vi "Append_Suffiix.vi"(1 "Results file":path) -> (0 "appended path":path)   [LabVIEW 2020]
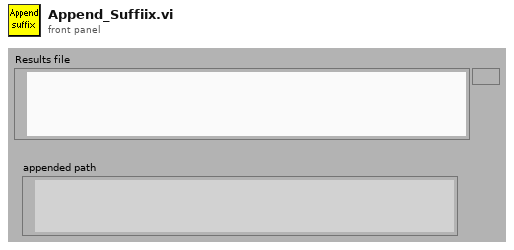
[diagram p1: front panel]
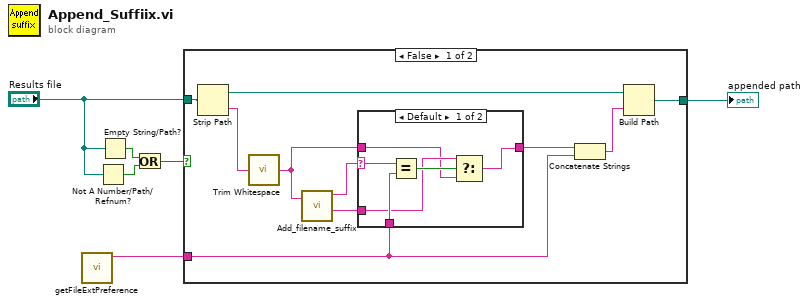
[diagram p0: block diagram]
diagram:
  n1 = call "getFileExtPreference.vi"() -> ("Suffix to add"=w1:string)  [unwired: 11 in]
  n2 = Not A Number/Path/Refnum?(number/path/refnum="Results file") -> (NaN/Path/Refnum?=w4:bool)
  n3 = Empty String/Path?(string/path="Results file") -> (empty?=w3:bool)
  n4 = Or(x=w3, y=w4) -> (x .or. y?=w2:bool)
  n5 = case shown="False" w2 {
    tunnel: [w16 w24] -> w6
    tunnel: "Results file" -> [w14 w24]
    tunnel: w1 -> [w8 _]
    frame False {
      n6 = Strip Path(path=w14) -> (stripped path=w15:path, name=w13:string)
      n7 = call <vilib>:"Trim Whitespace.vi"("string"=w13) -> ("trimmed string"=w9:string)  [unwired: 1 in]
      n8 = call "Add_filename_suffix.vi"("Filename"=w9) -> ("Original Suffix"=w12:string, "Base name"=w7:string)  [unwired: 1 in, 2 out]
      n9 = case shown="Default" w12 {
        selector: w12 -> [w21 _]
        tunnel: [w18 w23] -> w11
        tunnel: w7 -> [w19 w23]
        tunnel: w9 -> [w17 _]
        tunnel: w8 -> [w22 _]
        frame Default {
          n10 = Equal?(x=w21, y=w22) -> (x = y?=w20:bool)
          n11 = Select(t=w19, s=w20, f=w17) -> (s? t:f=w18:string)
        }
        frame ".csv", ".txt", ".xls" {
        }
      }
      n12 = Concatenate Strings(w11, w8) -> (w10:string)
      n13 = Build Path(base path=w15, name or relative path=w10) -> (appended path=w16:path)
    }
    frame True {
    }
  }
  "appended path" <- w6
